vi "Day 03 (Part Two).vi"() -> ()   [LabVIEW 2021]
panel:
  out "result":i32
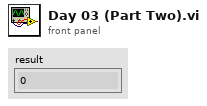
[diagram p1: front panel]
types:
  T1 = cluster{"number":i32, "start index":i32, "lenght":i32, "row":i32}
  T2 = cluster{"number":cluster{"number":i32, "start index":i32, "lenght":i32, "row":i32}, "columns":i32[], "rows":i32[]}
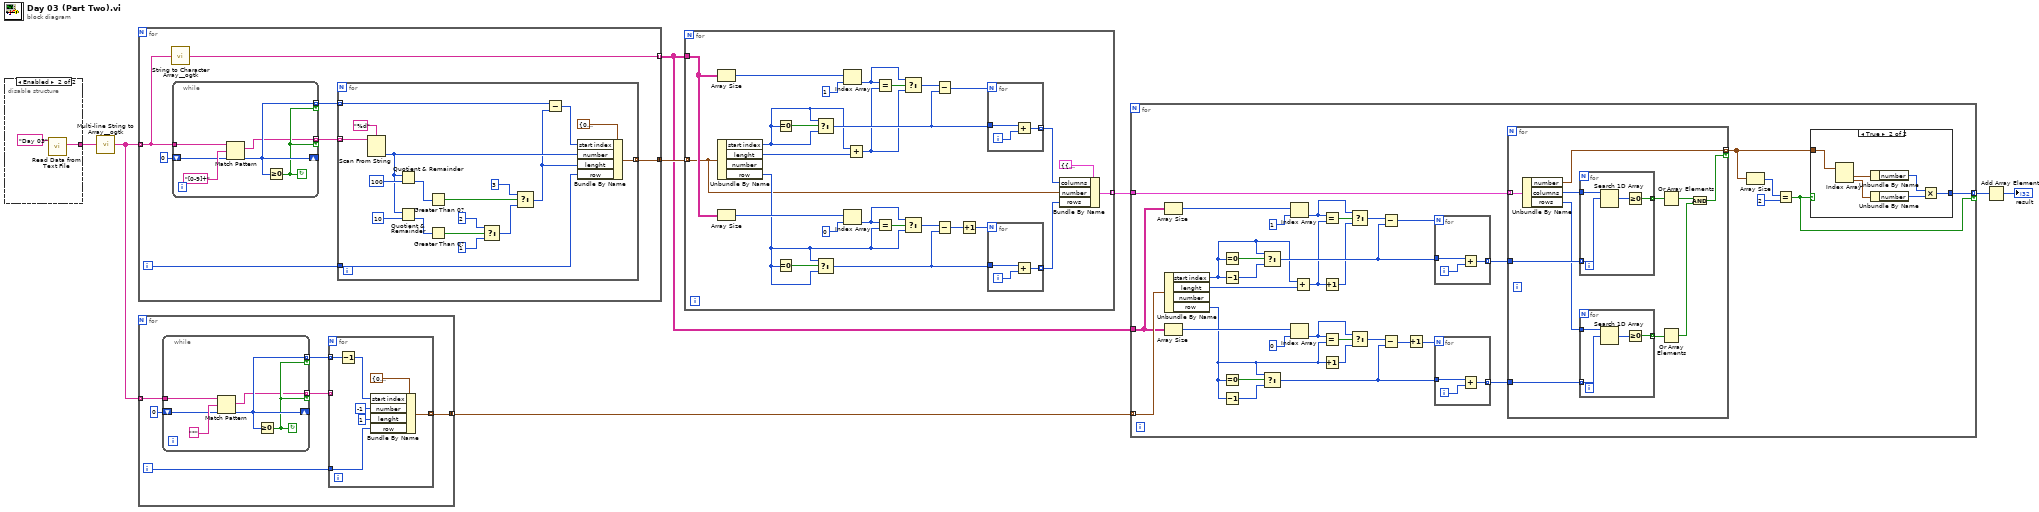
[diagram p0: block diagram]
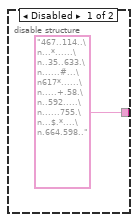
[diagram p2: hidden frame]
diagram:
  n1 = disable-structure shown="Enabled" {
    disable-tunnel: ["467..114..\n...*......\n..35..633.\n......#...\n617*......\n.....+.58.\n..592.....\n......755.\n...$.*....\n.664.598.." w11] -> w8
    frame Disabled {
    }
    frame Enabled {
      n2 = call "Read Data from Text File.vi"("Subfolder"="Day 03") -> ("data"=w11:string)  [unwired: 10 in]
    }
  }
  n3 = call <userlib>:"Multi-line String to Array__ogtk.vi"("string"=w8) -> ("lines"=w7:string[])
  n4 = for {
    tunnel: w7 -> [w14] mode=indexing
    tunnel: [w12] -> w6 mode=concatenating
    tunnel: [w13] -> w1 mode=indexing
    i -> [w15]
    n5 = call <userlib>:"String to Character Array__ogtk.vi"("Input String"=w14) -> ("Character Array"=w13:string[])
    n6 = while {
      tunnel: w14 -> [w43]
      shift-right: [w40] -> _
      shift-left: 0 ("offset past match") -> [w41]
      tunnel: [w38] -> w16 mode=indexing if=w39
      tunnel: [w40] -> w17 mode=indexing if=w39
      stop <- w39 continue-if-true
      n7 = Match Pattern(string=w43, regular expression="[0-9]+", offset (0)=w41) -> (match substring=w38:string, offset past match=w40:i32)  [unwired: 2 out]
      n8 = Greater Or Equal To 0?(x=w40) -> (x >= 0?=w39:bool)
    }
    n9 = for {
      tunnel: w17 -> [w21] mode=indexing
      tunnel: w16 -> [w36] mode=indexing
      tunnel: w15 -> [w34]
      tunnel: [w26] -> w12 mode=indexing
      n10 = Scan From String(format string="%d", input string=w36) -> (output 1=w25:i32)  [unwired: 3 in, 3 out]
      n11 = Quotient & Remainder(x=w25, y=100) -> (floor(x/y)=w27:i32)  [unwired: 1 out]
      n12 = Quotient & Remainder(x=w25, y=10) -> (floor(x/y)=w29:i32)  [unwired: 1 out]
      n13 = Greater Than 0?(x=w27) -> (x > 0?=w31:bool)
      n14 = Greater Than 0?(x=w29) -> (x > 0?=w30:bool)
      n15 = Select(t=2, s=w30, f=1) -> (s? t:f=w28:i32)
      n16 = Select(t=3, s=w31, f=w28) -> (s? t:f=w20:i32)
      n17 = Subtract(x=w21, y=w20) -> (x-y=w19:i32)
      n18 = Bundle By Name(cluster=T1 {"number"=0, "start index"=0, "lenght"=0, "row"=0}, "start index"=w19, "number"=w25, "lenght"=w20, "row"=w34) -> (w26:T1)
    }
  }
  n19 = for {
    tunnel: w7 -> [w45] mode=indexing
    tunnel: [w44] -> w5 mode=concatenating
    i -> [w46]
    n20 = while {
      tunnel: w45 -> [w62]
      shift-right: [w59] -> _
      shift-left: 0 ("offset past match") -> [w60]
      tunnel: [w57] -> w47 mode=indexing if=w58
      tunnel: [w59] -> w48 mode=indexing if=w58
      stop <- w58 continue-if-true
      n21 = Match Pattern(string=w62, regular expression="*", offset (0)=w60) -> (match substring=w57:string, offset past match=w59:i32)  [unwired: 2 out]
      n22 = Greater Or Equal To 0?(x=w59) -> (x >= 0?=w58:bool)
    }
    n23 = for {
      tunnel: w48 -> [w53] mode=indexing
      tunnel: w47 -> [_] mode=indexing
      tunnel: w46 -> [w55]
      tunnel: [w54] -> w44 mode=indexing
      n24 = Decrement(x=w53) -> (x-1=w52:i32)
      n25 = Bundle By Name(cluster=T1 {"number"=0, "start index"=0, "lenght"=0, "row"=0}, "start index"=w52, "number"=-1, "lenght"=1, "row"=w55) -> (w54:T1)
    }
  }
  n26 = for {
    tunnel: w6 -> [w66] mode=indexing
    tunnel: w1 -> [w71]
    tunnel: [w63] -> w4 mode=indexing
    n27 = Array Size(array=w71) -> (size(s)=w88:i32[])
    n28 = Unbundle By Name(w66) -> ("start index"=w70:i32, "lenght"=w86:i32, "row"=w68:i32)  [unwired: 1 out]
    n29 = Array Size(array=w71) -> (size(s)=w80:i32[])
    n30 = Equal To 0?(x=w70) -> (x = 0?=w89:bool)
    n31 = Equal To 0?(x=w68) -> (x = 0?=w79:bool)
    n32 = Select(t=w70, s=w89, f=w70) -> (s? t:f=w73:i32)
    n33 = Select(t=w68, s=w79, f=w68) -> (s? t:f=w72:i32)
    n34 = Index Array(array=w88, index=1) -> (element=w84:i32)
    n35 = Index Array(array=w80, index=0) -> (element=w83:i32)
    n36 = Add(x=w70, y=w86) -> (x+y=w69:i32)
    n37 = Equal?(x=w84, y=w69) -> (x = y?=w85:bool)
    n38 = Equal?(x=w83, y=w68) -> (x = y?=w82:bool)
    n39 = Select(t=w84, s=w85, f=w69) -> (s? t:f=w78:i32)
    n40 = Select(t=w83, s=w82, f=w68) -> (s? t:f=w74:i32)
    n41 = Subtract(x=w78, y=w73) -> (x-y=w77:i32)
    n42 = Subtract(x=w74, y=w72) -> (x-y=w75:i32)
    n43 = Increment(x=w75) -> (x+1=w76:i32)
    n44 = for {
      N: w77 -> [_]
      tunnel: w73 -> [w95]
      tunnel: [w93] -> w64 mode=indexing
      i -> [w94]
      n45 = Add(x=w95, y=w94) -> (x+y=w93:i32)
    }
    n46 = for {
      N: w76 -> [_]
      tunnel: w72 -> [w92]
      tunnel: [w90] -> w65 mode=indexing
      i -> [w91]
      n47 = Add(x=w92, y=w91) -> (x+y=w90:i32)
    }
    n48 = Bundle By Name(cluster=T2 {"number"={"number"=0, "start index"=0, "lenght"=0, "row"=0}, "columns"=[], "rows"=[]}, "columns"=w64, "number"=w66, "rows"=w65) -> (w63:T2)
  }
  n49 = for {
    tunnel: w5 -> [w130] mode=indexing
    tunnel: w1 -> [w111]
    tunnel: w4 -> [w101]
    tunnel: [w97] -> w3 mode=indexing if=w96
    n50 = Array Size(array=w111) -> (size(s)=w128:i32[])
    n51 = Unbundle By Name(w130) -> ("start index"=w110:i32, "lenght"=w126:i32, "row"=w108:i32)  [unwired: 1 out]
    n52 = Array Size(array=w111) -> (size(s)=w120:i32[])
    n53 = Equal To 0?(x=w110) -> (x = 0?=w129:bool)
    n54 = Decrement(x=w110) -> (x-1=w106:i32)
    n55 = Equal To 0?(x=w108) -> (x = 0?=w119:bool)
    n56 = Decrement(x=w108) -> (x-1=w107:i32)
    n57 = Select(t=w110, s=w129, f=w106) -> (s? t:f=w113:i32)
    n58 = Select(t=w108, s=w119, f=w107) -> (s? t:f=w112:i32)
    n59 = Index Array(array=w128, index=1) -> (element=w124:i32)
    n60 = Index Array(array=w120, index=0) -> (element=w123:i32)
    n61 = Add(x=w110, y=w126) -> (x+y=w109:i32)
    n62 = Equal?(x=w124, y=w109) -> (x = y?=w125:bool)
    n63 = Increment(x=w109) -> (x+1=w105:i32)
    n64 = Equal?(x=w123, y=w108) -> (x = y?=w122:bool)
    n65 = Increment(x=w108) -> (x+1=w104:i32)
    n66 = Select(t=w124, s=w125, f=w105) -> (s? t:f=w118:i32)
    n67 = Select(t=w123, s=w122, f=w104) -> (s? t:f=w114:i32)
    n68 = Subtract(x=w118, y=w113) -> (x-y=w117:i32)
    n69 = Subtract(x=w114, y=w112) -> (x-y=w115:i32)
    n70 = Increment(x=w115) -> (x+1=w116:i32)
    n71 = for {
      N: w117 -> [_]
      tunnel: w113 -> [w161]
      tunnel: [w159] -> w103 mode=indexing
      i -> [w160]
      n72 = Add(x=w161, y=w160) -> (x+y=w159:i32)
    }
    n73 = for {
      N: w116 -> [_]
      tunnel: w112 -> [w158]
      tunnel: [w156] -> w102 mode=indexing
      i -> [w157]
      n74 = Add(x=w158, y=w157) -> (x+y=w156:i32)
    }
    n75 = for {
      tunnel: w103 -> [w146]
      tunnel: w102 -> [w145]
      tunnel: w101 -> [w147] mode=indexing
      tunnel: [w140] -> w98 mode=indexing if=w139
      n76 = Unbundle By Name(w147) -> ("number"=w140:T1, "columns"=w138:i32[], "rows"=w137:i32[])
      n77 = for {
        tunnel: w146 -> [w154] mode=indexing
        tunnel: w138 -> [w155]
        tunnel: [w152] -> w144 mode=indexing
        n78 = Search 1D Array(1D array=w155, element=w154) -> (index of element=w153:i32)  [unwired: 1 in]
        n79 = Greater Or Equal To 0?(x=w153) -> (x >= 0?=w152:bool)
      }
      n80 = for {
        tunnel: w145 -> [w150] mode=indexing
        tunnel: w137 -> [w151]
        tunnel: [w148] -> w143 mode=indexing
        n81 = Search 1D Array(1D array=w151, element=w150) -> (index of element=w149:i32)  [unwired: 1 in]
        n82 = Greater Or Equal To 0?(x=w149) -> (x >= 0?=w148:bool)
      }
      n83 = Or Array Elements(Boolean array=w144) -> (logical OR=w141:bool)
      n84 = Or Array Elements(Boolean array=w143) -> (logical OR=w142:bool)
      n85 = And(x=w141, y=w142) -> (x .and. y?=w139:bool)
    }
    n86 = Array Size(array=w98) -> (size(s)=w100:i32)
    n87 = Equal?(x=w100, y=2) -> (x = y?=w96:bool)
    n88 = case shown="True" w96 {
      tunnel: w98 -> [_ w136]
      tunnel: [_ w131] -> w97
      frame False {
      }
      frame True {
        n89 = Index Array(array=w136) -> (element #1=w135:T1, element #2=w134:T1)  [unwired: 2 in]
        n90 = Unbundle By Name(w135) -> ("number"=w133:i32)
        n91 = Unbundle By Name(w134) -> ("number"=w132:i32)
        n92 = Multiply(x=w133, y=w132) -> (x*y=w131:i32)
      }
    }
  }
  n93 = Add Array Elements(numeric array=w3) -> (sum=→"result":i32)
